vi "Upper Case & Lower Case.vi"() -> ()   [LabVIEW 2016]
panel:
  out "Upper Case":string
  out "Lower Case":string
  in  "Upper Case":string
  in  "Lower Case":string
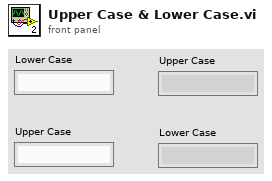
[diagram p1: front panel]
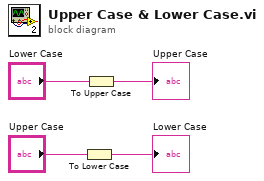
[diagram p0: block diagram]
diagram:
  n1 = To Lower Case(string="Upper Case") -> (all lower case string=→"Lower Case":string)
  n2 = To Upper Case(1:"Lower Case") -> (0:→"Upper Case":string)
